vi "PROGRAMA6_QUIZ.vi"() -> ()   [LabVIEW 2013]
panel:
  out "ACEPTADO":bool
  out "EDAD":dbl
  in  "EXPERIENCIA":u16(ring) items=["EXPERIENCIA", "NO TIENE EXPERIENCIA"]
  in  "TIENE TITULO":u16(ring) items=["NO TIENE", "SI TIENE"]
  # "SE DEBE DE SELECCIONAR SI TIENE O NO TIENE TITULO,\nLUEGO SI TIENE EXPERIENCIA Y GENERAR LA EDAD ENTRE \n20-70.\nES CONTRATADO SI LA EDAD ES MAYOR A 25 Y SI TIENE \nEXPERIENCIA O SI TIENE TITULO Y NO TIENE EXPERIENCIA\nY ES MAYOR A 25"
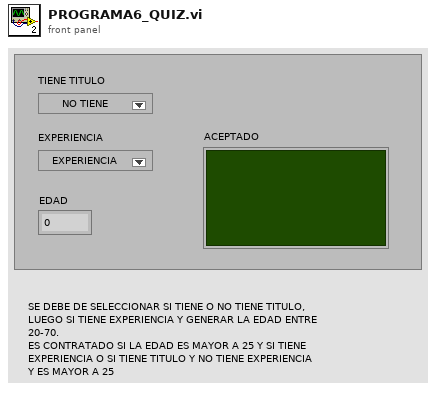
[diagram p1: front panel]
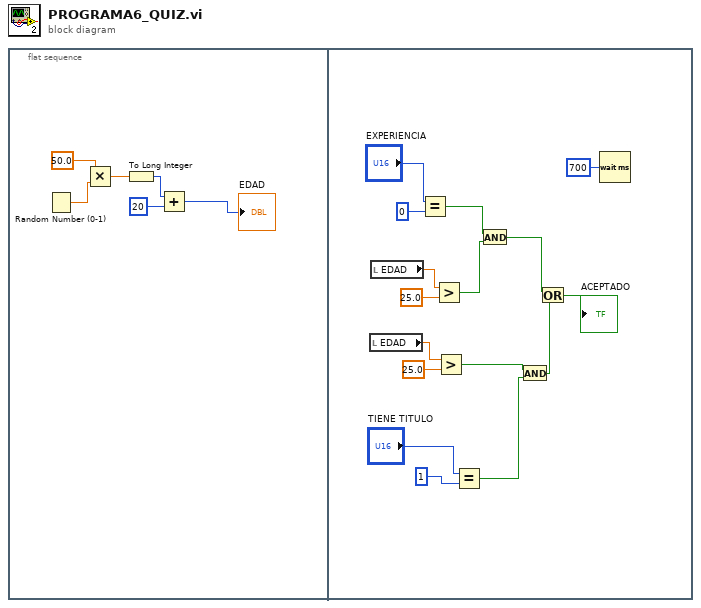
[diagram p0: block diagram]
diagram:
  n1 = flat-sequence {
    frame #0 {
      n2 = Random Number (0-1)() -> (number: 0 to 1=w5:dbl)
      n3 = Multiply(x=50.0, y=w5) -> (x*y=w4:dbl)
      n4 = To Long Integer(number=w4) -> (32bit integer=w3:i32)
      n5 = Add(x=w3, y=20) -> (x+y=→"EDAD":i32)
    }
    frame #1 {
      n6 = local read "EDAD"() -> (w17:dbl)
      n7 = local read "EDAD"() -> (w20:dbl)
      n8 = Equal?(x="EXPERIENCIA", y=u16 0) -> (x = y?=w14:bool)
      n9 = Greater?(x=w20, y=25.0) -> (0:w13:bool)
      n10 = Greater?(x=w17, y=25.0) -> (0:w11:bool)
      n11 = Equal?(x="TIENE TITULO", y=u16 1) -> (x = y?=w10:bool)
      n12 = And(x=w14, y=w13) -> (x .and. y?=w12:bool)
      n13 = And(x=w11, y=w10) -> (x .and. y?=w9:bool)
      n14 = Or(x=w12, y=w9) -> (x .or. y?=→"ACEPTADO":bool)
      n15 = Wait (ms)(milliseconds to wait=u32 700) -> ()  [unwired: 1 out]
    }
  }
